vi "PH_SRDG645.PC Set Channel.vi"(0 "i ref in":refnum<vi>, 1 "Channel to set":T1 items=["T0", "T1", "A", "B", "C", "D", "E", "F", "G", "H"], 2 "Channel Settings":T2={"Delay [s]"=0.0, "relative to"=1000} {"relative to" items=["T0", "T1", "A", "B", "C", "D", "E", "F", "G", "H"]; "Delay [s]" format="%#_12p"}, 5 "error IO":errorcluster) -> (14 "i ref out":refnum<vi>, 17 "Something changed?":bool, 19 "error out":errorcluster)   [LabVIEW 2014, in "PH_SRDG645.lvlib"]
doc: "This VI communicates with the hardware to set the channel settings."
uses:
  PH_SRDG645.lvlib
  PH_SRDG645.Channel Settings.ctl
  instr.lib/SRDG645/Driver/Channel.ctl
  instr.lib/SRDG645/Stanford Research DG645 - Driver.lvlib
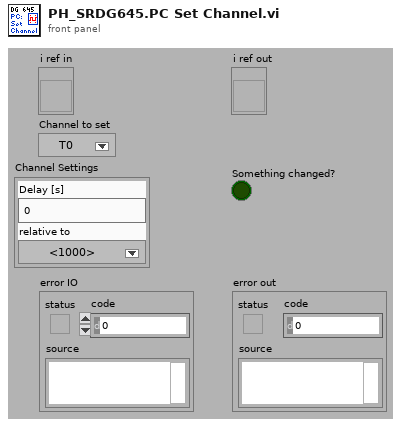
[diagram p1: front panel]
types:
  T1 = typedef "Stanford Research DG645 - Driver.lvlib/Channel.ctl" = i32
  T2 = typedef "PH_SRDG645.lvlib/PH_SRDG645.Channel Settings.ctl" = cluster{"Delay [s]":dbl, "relative to":i32}
  T3 = typedef "PH_SRDG645.lvlib/PH_SRDG645.i attribute.ctl" = cluster{"GUI Refs":cluster{"Delete":refnum<vi>, "Device Errors":refnum<vi>, "Trigger":refnum<vi>, "Default Name":refnum<vi>, "Firmware Revision":refnum<vi>, "Serial Number":refnum<vi>, "Model":refnum<vi>, "Visa resource name":refnum<vi>}, "Service ID Rate":i32, "Service IDs Channelinfo":i32[], "VISA resource name":refnum<visa-resource-name>, "Device Errors":cluster{"code":i32, "Text":string}[], "Trigger":T4, "Channels":cluster{"T1":T2, "A":T2, "B":T2, "C":T2, "D":T2, "E":T2, "F":T2, "G":T2, "H":T2}, "GUI Refs Channels":refnum<vi>[], "Outputs":cluster{"AB":cluster{"Level Offset [V]":dbl, "Amplitue [V]":dbl, "Polarity":i32}, "CD":cluster{"Level Offset [V]":dbl, "Amplitue [V]":dbl, "Polarity":i32}, "EF":cluster{"Level Offset [V]":dbl, "Amplitue [V]":dbl, "Polarity":i32}, "GH":cluster{"Level Offset [V]":dbl, "Amplitue [V]":dbl, "Polarity":i32}, "T0":cluster{"Level Offset [V]":dbl, "Amplitue [V]":dbl, "Polarity":i32}}, "GUI Refs Outputs":refnum<vi>[], "Serial Number":string, "Firmweare Revision":string, "Model":string}
  T4 = typedef "PH_SRDG645.lvlib/PH_SRDG645.Trigger.ctl" = cluster{"Source":i32, "Rate [Hz]":dbl, "Level [V]":dbl}
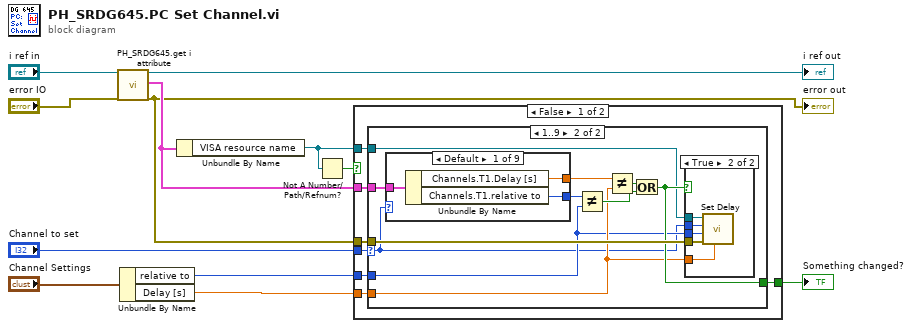
[diagram p0: block diagram]
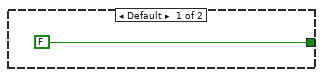
[diagram p2: hidden frame]
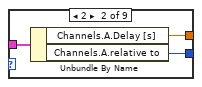
[diagram p3: hidden frame]
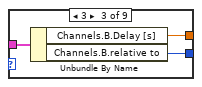
[diagram p4: hidden frame]
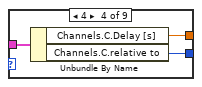
[diagram p5: hidden frame]
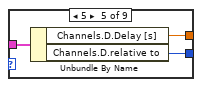
[diagram p6: hidden frame]
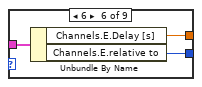
[diagram p7: hidden frame]
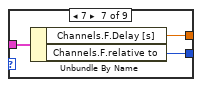
[diagram p8: hidden frame]
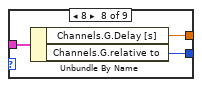
[diagram p9: hidden frame]
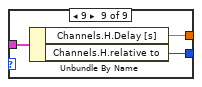
[diagram p10: hidden frame]
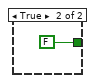
[diagram p12: hidden frame]
diagram:
  n1 = call "PH_SRDG645.get i attribute.vi"("i ref in"="i ref in", "error in (no error)"="error IO") -> ("i ref out"=→"i ref out":refnum<vi>, "i attribute"=w4:T3, "error out"=w1:errorcluster)  [unwired: 15 in]
  "error out" <- w1
  n2 = Unbundle By Name("Channel Settings") -> ("relative to"=w8:i32, "Delay [s]"=w7:dbl)
  n3 = Unbundle By Name(w4) -> ("VISA resource name"=w3:refnum<visa-resource-name>)
  n4 = Not A Number/Path/Refnum?(number/path/refnum=w3) -> (NaN/Path/Refnum?=w2:bool)
  n5 = case shown="False" w2 {
    tunnel: w1 -> [w19 _]
    tunnel: w8 -> [w18 _]
    tunnel: w7 -> [w17 _]
    tunnel: [w16 FALSE] -> w6
    tunnel: "Channel to set" -> [w15 _]
    tunnel: w4 -> [w14 _]
    tunnel: w3 -> [w13 _]
    frame False {
      n6 = case shown="1..9" w15 {
        selector: w15 -> [_ w22]
        tunnel: w14 -> [_ w31]
        tunnel: w19 -> [_ w30]
        tunnel: w18 -> [_ w23]
        tunnel: w17 -> [_ w24]
        tunnel: [FALSE w25] -> w16
        tunnel: w13 -> [_ w21]
        frame Default {
        }
        frame 1..9 {
          n7 = case shown="Default" w22 {
            tunnel: w31 -> [w34 w37 w40 w43 w46 w49 w52 w55 w58]
            tunnel: [w33 w36 w39 w42 w45 w48 w51 w54 w57] -> w29
            tunnel: [w32 w35 w38 w41 w44 w47 w50 w53 w56] -> w28
            frame Default {
              n8 = Unbundle By Name(w34) -> ("Channels.T1.Delay [s]"=w32:dbl, "Channels.T1.relative to"=w33:i32)
            }
            frame 2 {
              n9 = Unbundle By Name(w37) -> ("Channels.A.Delay [s]"=w35:dbl, "Channels.A.relative to"=w36:i32)
            }
            frame 3 {
              n10 = Unbundle By Name(w40) -> ("Channels.B.Delay [s]"=w38:dbl, "Channels.B.relative to"=w39:i32)
            }
            frame 4 {
              n11 = Unbundle By Name(w43) -> ("Channels.C.Delay [s]"=w41:dbl, "Channels.C.relative to"=w42:i32)
            }
            frame 5 {
              n12 = Unbundle By Name(w46) -> ("Channels.D.Delay [s]"=w44:dbl, "Channels.D.relative to"=w45:i32)
            }
            frame 6 {
              n13 = Unbundle By Name(w49) -> ("Channels.E.Delay [s]"=w47:dbl, "Channels.E.relative to"=w48:i32)
            }
            frame 7 {
              n14 = Unbundle By Name(w52) -> ("Channels.F.Delay [s]"=w50:dbl, "Channels.F.relative to"=w51:i32)
            }
            frame 8 {
              n15 = Unbundle By Name(w55) -> ("Channels.G.Delay [s]"=w53:dbl, "Channels.G.relative to"=w54:i32)
            }
            frame 9 {
              n16 = Unbundle By Name(w58) -> ("Channels.H.Delay [s]"=w56:dbl, "Channels.H.relative to"=w57:i32)
            }
          }
          n17 = Not Equal?(x=w29, y=w23) -> (x != y?=w26:bool)
          n18 = Not Equal?(x=w28, y=w24) -> (x != y?=w27:bool)
          n19 = Or(x=w27, y=w26) -> (x .or. y?=w25:bool)
          n20 = case shown="True" w25 {
            tunnel: w23 -> [_ w62]
            tunnel: w21 -> [_ w63]
            tunnel: w30 -> [_ w59]
            tunnel: w24 -> [_ w61]
            tunnel: w22 -> [_ w60]
            frame False {
            }
            frame True {
              n21 = call "Set Delay.vi"("Delay (0) [s]"=w61, "error in (no error)"=w59, "relative to (T0)"=w62, "Channel (T0)"=w60, "VISA resource name"=w63) -> ()  [unwired: 4 in, 3 out]
            }
          }
        }
      }
    }
    frame True {
    }
  }
  "Something changed?" <- w6
